vi "Set Offset.vi"(6 "Channel":i32=1, 8 "error in (no error)":errorcluster, 10 "Offset":dbl, 11 "336XX in":refnum<class "336XX.lvclass">) -> (0 "error out":errorcluster, 3 "336XX out":refnum<class "336XX.lvclass">)   [LabVIEW 2019, in "336XX.lvlib" / "336XX.lvclass"]
uses:
  Library/336XX.lvclass
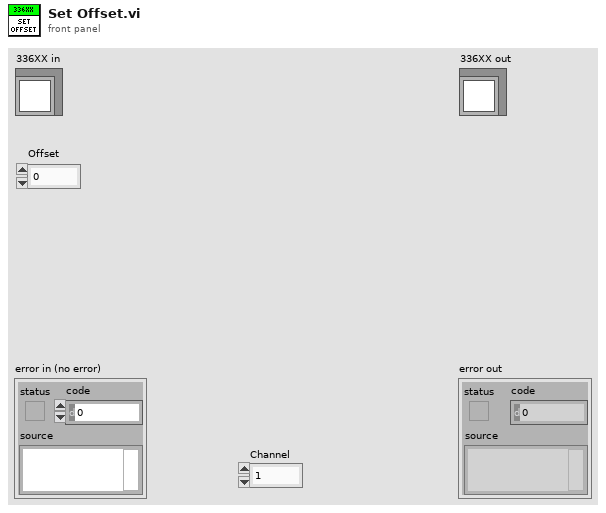
[diagram p1: front panel]
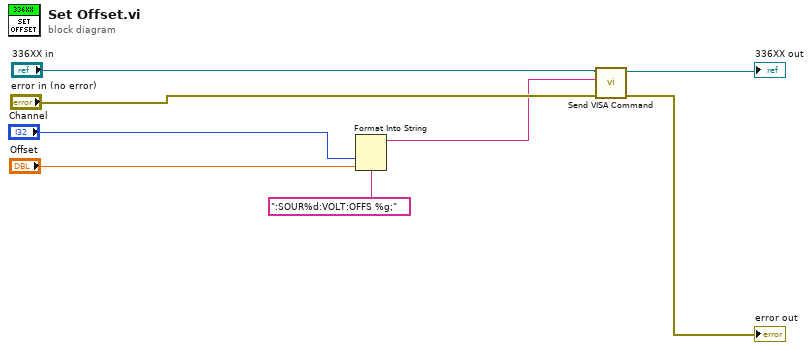
[diagram p0: block diagram]
diagram:
  n1 = Format Into String(format string=":SOUR%d:VOLT:OFFS %g;", "Channel", "Offset") -> (resulting string=w3:string)  [unwired: 2 in, 1 out]
  n2 = call "Send VISA Command.vi"("error in (no error)"="error in (no error)", "Command"=w3, "336XX in"="336XX in") -> ("error out"=→"error out":errorcluster, "336XX out"=→"336XX out":refnum<class "336XX.lvclass">)  [unwired: 7 in]
